vi "ParseControlPath.vi"(5 "VI":refnum<vi>, 8 "error in (no error)":errorcluster, 10 "control path string":string, 11 "Controls[]":refnum<vi>[](array[refnum])) -> (0 "error out":errorcluster, 1 "value element":refnum<vi>, 2 "subcontrol path":T1(array[cluster]), 3 "control":refnum<vi>)   [LabVIEW 2021, in "SetGetControlValue.lvlib"]
uses:
  SetGetControlValue.lvlib
  <vilib>/regexp/Match Regular Expression.xnode
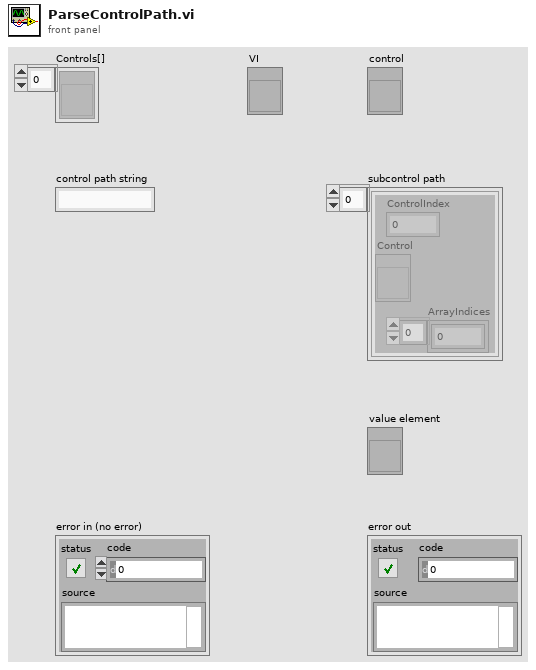
[diagram p1: front panel]
types:
  T1 = cluster{"ControlIndex":i32, "Control":refnum<vi>, "ArrayIndices":i32[]}[]
  T2 = cluster{"ControlIndex":i32, "Control":refnum<vi>, "ArrayIndices":i32[]}
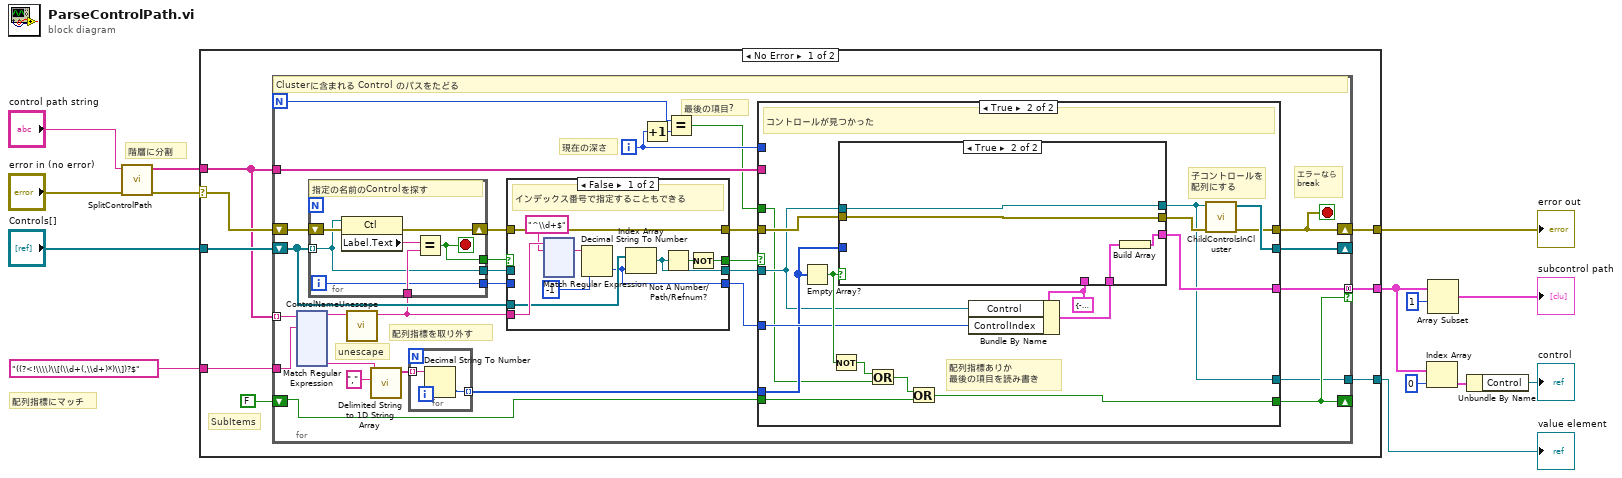
[diagram p0: block diagram]
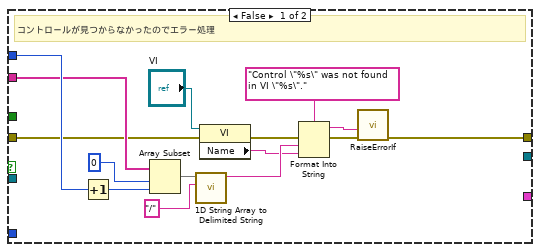
[diagram p3: hidden frame]
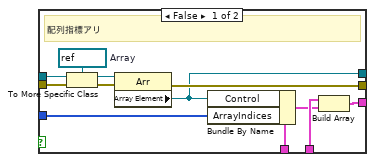
[diagram p4: hidden frame]
diagram:
  # "階層に分割"
  # "配列指標にマッチ"
  n1 = call "SplitControlPath.vi"("error in"="error in (no error)", "control path string"="control path string") -> ("error out"=w2:errorcluster, "string array"=w1:string[])  [unwired: 8 in]
  n2 = case shown="No Error" w2 {
    selector: w2 -> [w16 w360]
    tunnel: [w22 w360] -> w14
    tunnel: "Controls[]" -> [w20 _]
    tunnel: "((?<!\\\\)\\[(\\d+(,\\d+)*)\\])?$" ("regular expression") -> [w19 _]
    tunnel: [w18 _] -> w9
    tunnel: [w17 _] -> w5
    tunnel: w1 -> [w15 _]
    frame No Error {
      # "SubItems"
      n3 = for {
        N -> [w29]
        tunnel: w15 -> [w49] mode=indexing
        shift-right: [w51] -> _
        shift-left: w20 -> [w41]
        shift-right: [w43] -> w22
        shift-left: w16 -> [w50]
        tunnel: w15 -> [w44]
        shift-right: [w27] -> _
        shift-left: FALSE -> [w25]
        tunnel: w19 -> [w33]
        tunnel: [w32] -> w18 mode=concatenating if=w27
        tunnel: [w26] -> w17
        i -> [w31]
        stop <- w43 stop-if-true
        # "unescape"
        # "最後の項目?"
        # "現在の深さ"
        # "エラーなら\nbreak"
        # "配列指標を取り外す"
        # "Clusterに含まれる Control のパスをたどる"
        n4 = xnode "Match Regular Expression"("input string"=w49, "regular expression"=w33) -> ("before match"=w24:string, "submatch 2"=w48:string)  [unwired: 4 in, 5 out]
        n5 = call "ControlNameUnescape.vi"("escaped string"=w24) -> ("label"=w23:string)  [unwired: 10 in]
        n6 = for {
          tunnel: w41 -> [w307] mode=indexing
          tunnel: w23 -> [w308]
          shift-right: [w310] -> w38
          shift-left: w50 -> [w311]
          tunnel: [w307] -> w36
          tunnel: [w306] -> w42
          tunnel: [w305] -> w35
          i -> [w305]
          stop <- w306 stop-if-true
          # "指定の名前のControlを探す"
          n7 = property class="Ctl"(reference=w307, error in=w311) -> (error out=w310:errorcluster, "Label.Text"=w309:string)  [unwired: 1 out]
          n8 = Equal?(x=w309, y=w308) -> (x = y?=w306:bool)
        }
        n9 = call <vilib>:"Delimited String to 1D String Array.vi"("delimiter"=",", "delimited string"=w48) -> ("string array"=w46:string[])  [unwired: 9 in]
        n10 = for {
          tunnel: w46 -> [w184] mode=indexing
          tunnel: [w183] -> w45 mode=indexing
          n11 = Decimal String To Number(string=w184) -> (number=w183:i32)  [unwired: 2 in, 1 out]
        }
        n12 = case shown="False" w42 {
          selector: w42 -> [_ w182]
          tunnel: w23 -> [w61 _]
          tunnel: w41 -> [w57 _]
          tunnel: [w56 w182] -> w40
          tunnel: [w53 w181] -> w39
          tunnel: w38 -> [w53 w181]
          tunnel: [w54 w180] -> w37
          tunnel: w36 -> [_ w180]
          tunnel: w35 -> [_ w179]
          tunnel: [w52 w179] -> w34
          frame False {
            # "インデックス番号で指定することもできる"
            n13 = xnode "Match Regular Expression"("input string"=w61, "regular expression"="^\\d+$") -> ("whole match"=w59:string)  [unwired: 4 in, 4 out]
            n14 = Decimal String To Number(string=w59, default (0L)=-1 ("default (0 I32)")) -> (number=w52:i32)  [unwired: 1 in, 1 out]
            n15 = Index Array(array=w57, index=w52) -> (element=w54:refnum<vi>)
            n16 = Not A Number/Path/Refnum?(number/path/refnum=w54) -> (NaN/Path/Refnum?=w55:bool)
            n17 = Not(x=w55) -> (.not. x?=w56:bool)
          }
          frame True {
            # "見つかった"
          }
        }
        n18 = Increment(x=w31) -> (x+1=w30:i32)
        n19 = Equal?(x=w29, y=w30) -> (x = y?=w28:bool)
        n20 = case shown="True" w40 {
          tunnel: [_ w343] -> w51
          tunnel: [w316 w340] -> w43
          tunnel: w37 -> [_ w331]
          tunnel: w39 -> [w312 w341]
          tunnel: w45 -> [_ w336]
          tunnel: w44 -> [w318 _]
          tunnel: w31 -> [w324 _]
          tunnel: w34 -> [_ w338]
          tunnel: w25 -> [_ w332]
          tunnel: [_ w333] -> w27
          tunnel: [_ w334] -> w32
          tunnel: w28 -> [_ w329]
          tunnel: [_ w327] -> w26
          frame False {
            # "コントロールが見つからなかったのでエラー処理"
            n21 = Increment(x=w324) -> (x+1=w325:i32)
            n22 = Array Subset(array=w318, index=0, length=w325) -> (w323:string[])
            n23 = call <vilib>:"1D String Array to Delimited String.vi"("delimiter"="/", "string array"=w323) -> ("delimited string"=w321:string)  [unwired: 9 in]
            n24 = property class="VI"(reference="VI", error in=w312) -> (error out=w315:errorcluster, "Name"=w319:string)  [unwired: 1 out]
            n25 = Format Into String(format string="Control \"%s\" was not found in VI \"%s\".", error in=w315, w321, w319) -> (resulting string=w317:string, error out=w314:errorcluster)  [unwired: 1 in]
            n26 = call "RaiseErrorIf.vi"("error in (no error)"=w314, "error message"=w317) -> ("error out"=w316:errorcluster)  [unwired: 9 in]
          }
          frame True {
            w335 = T2 {"ControlIndex"=-1, "Control"=refnum, "ArrayIndices"=[]}
            # "配列指標ありか\n最後の項目を読み書き"
            # "子コントロールを\n配列にする"
            # "コントロールが見つかった"
            n27 = Empty Array?(array=w336) -> (empty?=w339:bool)
            n28 = Not(x=w339) -> (.not. x?=w330:bool)
            n29 = Or(x=w330, y=w329) -> (x .or. y?=w328:bool)
            n30 = Or(x=w328, y=w332) -> (x .or. y?=w333:bool)
            n31 = Bundle By Name(cluster=w335, "Control"=w331, "ControlIndex"=w338) -> (w337:T2)
            n32 = case shown="True" w339 {
              tunnel: w331 -> [w354 w358]
              tunnel: [w349 w358] -> w327
              tunnel: [w351 w359] -> w342
              tunnel: w341 -> [w350 w359]
              tunnel: w337 -> [w347 w357]
              tunnel: w336 -> [w348 _]
              tunnel: w335 -> [w345 _]
              tunnel: [w344 w356] -> w334
              frame False {
                w355 = refnum<vi> refnum  # Array
                # "配列指標アリ"
                n33 = To More Specific Class(target class=w355, reference=w354, error in=w350) -> (specific class reference=w353:refnum<vi>, error out=w352:errorcluster)
                n34 = property class="Arr"(reference=w353, error in=w352) -> (error out=w351:errorcluster, "Array Element"=w349:refnum<vi>)  [unwired: 1 out]
                n35 = Bundle By Name(cluster=w345, "Control"=w349, "ArrayIndices"=w348) -> (w346:T2)
                n36 = Build Array(w347, w346) -> (w344:T1)
              }
              frame True {
                n37 = Build Array(w357) -> (w356:T1)
              }
            }
            n38 = call "ChildControlsInCluster.vi"("error in (no error)"=w342, "Control in"=w327) -> ("error out"=w340:errorcluster, "Controls[]"=w343:refnum<vi>[])  [unwired: 7 in, 1 out]
          }
        }
      }
    }
    frame Error {
    }
  }
  "error out" <- w14
  "value element" <- w5
  n39 = Index Array(array=w9, index=0) -> (element=w7:T2)
  n40 = Array Subset(array=w9, index=1) -> (→"subcontrol path":T1)  [unwired: 1 in]
  n41 = Unbundle By Name(w7) -> ("Control"=→"control":refnum<vi>)
